vi "Main.vi"() -> ()   [LabVIEW 2015]
doc: "The myRIO Project template acquires acceleration data from the onboard accelerometer and displays the changes of acceleration values in a waveform chart."
uses:
  <vilib>/myRIO/Common/Instrument Driver Framework/myRIO v1.0/Encoder/typedefs/Encoder Signal Mode.ctl
  <vilib>/myRIO/Instrument Drivers/Onboard IO/Encoder/typedefs/Encoder Reference.ctl
  <vilib>/myRIO/Common/Instrument Driver Framework/Utilities/typedefs/myRIO Generic Hardware Reference.ctl
  <vilib>/myRIO/Common/Instrument Driver Framework/Utilities/typedefs/Hardware Version Enum.ctl
  <vilib>/myRIO/Common/Instrument Driver Framework/Utilities/typedefs/myRIO v1.0 Reference.ctl
  <vilib>/myRIO/Common/Instrument Driver Framework/Utilities/typedefs/Generic FPGA Reference.ctl
  <vilib>/myRIO/Common/Instrument Driver Framework/myRIO v1.0/Encoder/typedefs/Encoder Channels Enum.ctl
  <vilib>/myRIO/Common/Instrument Driver Framework/myRIO v1.0/Encoder/typedefs/Encoder Configuration v1.0.ctl
  <vilib>/userdefined/High Color/nirio_resource_hc.ctl
  <vilib>/myRIO/Instrument Drivers/Onboard IO/PWM/typedefs/PWM Reference.ctl
  <vilib>/myRIO/Common/Instrument Driver Framework/myRIO v1.0/PWM/typedefs/PWM Channels Enum.ctl
  <vilib>/myRIO/Instrument Drivers/Onboard IO/PWM/typedefs/PWM Configuration.ctl
  <vilib>/myRIO/Instrument Drivers/Onboard IO/DIO/typedefs/DIO Reference.ctl
  <vilib>/myRIO/Common/Instrument Driver Framework/myRIO v1.0/DIO/typedefs/DIO Channels List.ctl
  <vilib>/myRIO/Common/Instrument Driver Framework/myRIO v1.0/DIO/typedefs/DIO Channels Enum.ctl
  <vilib>/myRIO/Common/Instrument Driver Framework/Utilities/vis/Is FPGA Ref Available.vi
  <vilib>/myRIO/Common/Instrument Driver Framework/myRIO v1.0/Encoder/vis/myRIO v1.1 Open Encoder.vi
  <vilib>/myRIO/Instrument Drivers/Onboard IO/Encoder/vis/Read.vi
  <vilib>/myRIO/Common/Instrument Driver Framework/myRIO v1.0/PWM/vis/myRIO v1.1 Open PWM.vi
  <vilib>/myRIO/Instrument Drivers/Onboard IO/PWM/vis/Set Duty Cycle and Frequency.vi
  <vilib>/myRIO/Common/Instrument Driver Framework/myRIO v1.0/DIO/vis/myRIO v1.1 Open DIO.vi
  <vilib>/myRIO/Instrument Drivers/Onboard IO/DIO/vis/Write.vi
  <vilib>/myRIO/Common/Instrument Driver Framework/Utilities/vis/Validate Channels.vi
  <vilib>/myRIO/Common/Instrument Driver Framework/myRIO v1.0/Encoder/vis/myRIO v1.0 Reserve Encoder.vi
  <vilib>/myRIO/Common/Instrument Driver Framework/myRIO v1.0/PWM/vis/myRIO v1.0 Reserve PWM.vi
  <vilib>/myRIO/Common/Instrument Driver Framework/myRIO v1.0/DIO/vis/myRIO v1.0 Reserve DIO.vi
  <vilib>/myRIO/Common/Instrument Driver Framework/myRIO v1.0/UART/vis/myRIO v1.0 Close UART.vi
  <vilib>/myRIO/Common/Instrument Driver Framework/myRIO v1.0/Encoder/vis/myRIO v1.0 Build MUX Configuration Encoder.vi
  <vilib>/myRIO/Common/Instrument Driver Framework/myRIO v1.0/Resource Manager/vis/myRIO v1.0 Reserve Channel List.vi
  <vilib>/myRIO/Common/Instrument Driver Framework/myRIO v1.0/PWM/vis/myRIO v1.0 Build MUX Configuration PWM.vi
  <vilib>/myRIO/Common/Instrument Driver Framework/myRIO v1.0/DIO/vis/myRIO v1.0 Build MUX Configuration DIO.vi
  <vilib>/myRIO/Common/Instrument Driver Framework/myRIO v1.0/Resource Manager/vis/myRIO v1.0 Create Configuration List.vi
  <vilib>/myRIO/Common/Instrument Driver Framework/myRIO v1.0/Resource Manager/vis/myRIO v1.0 Reserve Channel.vi
  <vilib>/myRIO/Common/Instrument Driver Framework/myRIO v1.0/Resource Manager/vis/myRIO v1.0 Unreserve Channel.vi
  <vilib>/myRIO/Common/Instrument Driver Framework/myRIO v1.0/Resource Manager/vis/myRIO v1.0 Build Mutex Name.vi
  <vilib>/Utility/VariantDataType/GetNumericInfo.vi
  <vilib>/Utility/error.llb/Error Cluster From Error Code.vi
  <vilib>/myRIO/Common/Instrument Driver Framework/myRIO v1.0/myRIO v1.1 Open.vi
  <vilib>/myRIO/Common/Instrument Driver Framework/Utilities/vis/IO Manager.vi
  <vilib>/myRIO/Common/Instrument Driver Framework/Utilities/vis/Configuration Manager.vi
  <vilib>/myRIO/Common/Instrument Driver Framework/myRIO v1.0/Resource Manager/vis/myRIO v1.0 Configure IO.vi
  <vilib>/myRIO/Common/Instrument Driver Framework/myRIO v1.0/myRIO v1.0 Close.vi
  <vilib>/myRIO/Common/Instrument Driver Framework/myRIO v1.0/Encoder/vis/myRIO v1.0 Configure Encoder.vi
  <vilib>/myRIO/Common/Instrument Driver Framework/myRIO v1.0/Encoder/vis/myRIO v1.0 Read Encoder.vi
  <vilib>/myRIO/Common/Instrument Driver Framework/myRIO v1.0/PWM/vis/myRIO v1.0 Write PWM.vi
  <vilib>/myRIO/Common/Instrument Driver Framework/myRIO v1.0/DIO/vis/myRIO v1.0 Write DIO.vi
  <vilib>/myRIO/Common/Instrument Driver Framework/Utilities/vis/FPGA Ref Manager.vi
  <vilib>/myRIO/Common/Instrument Driver Framework/myRIO v1.0/myRIO v1.0 Reset FPGA.vi
  <vilib>/myRIO/Common/Instrument Driver Framework/myRIO v1.0/IRQ/vis/myRIO v1.0 IRQ Info FGV.vi
  <vilib>/myRIO/Common/Instrument Driver Framework/myRIO v1.0/IRQ/vis/myRIO v1.0 Timer IRQ Info FGV.vi
  <vilib>/myRIO/Common/Instrument Driver Framework/myRIO v1.0/IRQ/vis/myRIO v1.0 ISR Agent.vi
  <vilib>/myRIO/Express VI/Onboard IO/Encoder/Encoder Express VI.xnode
  <vilib>/myRIO/Common/Instrument Driver Framework/myRIO v1.0/Encoder/typedefs/Encoder Count Direction Enum.ctl
  <vilib>/myRIO/Instrument Drivers/Onboard IO/Encoder/vis/myRIO Encoder Open.xnode
  <vilib>/myRIO/Express VI/Onboard IO/PWM/PWM Express VI.xnode
  <vilib>/myRIO/Instrument Drivers/Onboard IO/PWM/vis/myRIO PWM Open.xnode
  <vilib>/myRIO/Express VI/Onboard IO/DO/DO Express VI.xnode
  <vilib>/myRIO/Instrument Drivers/Onboard IO/DIO/vis/myRIO DIO Open.xnode
  <vilib>/myRIO/Instrument Drivers/Utilities/Utilities.lvlib
  <vilib>/myRIO/Instrument Drivers/Onboard IO/Encoder/Encoder.lvlib
  <vilib>/myRIO/Instrument Drivers/Onboard IO/DIO/DIO.lvlib
  <vilib>/myRIO/Instrument Drivers/Onboard IO/PWM/PWM.lvlib
panel:
  in  "Up/Down control":bool
  out "PWM":dbl(graph)
  in  "K4":dbl
  in  "K3":dbl
  in  "K2":dbl
  in  "K1":dbl
  in  "Stop Button":bool
  out "Gauge":dbl(knob) scale=0.0..360.0
  in  "ON OFF":bool
  out "x >= 0?":bool
  out ".not. x?":bool
  out "abs(x)":dbl
  out "filtTheta":dbl
  out "Theta control 2":dbl
  out "Theta control":dbl
  out "Control":bool
  out "dPhi":dbl(graph)
  out "dTheta":dbl(graph)
  in  "Swing up gain":dbl
  out "Rad dPhi":dbl
  out "Rad Theta":dbl
  out "Rad Phi":dbl
  out "Direction Motor":dbl
  out "Counter Motor":dbl
  out "error out":errorcluster
  # "Overview: The myRIO Project template acquires acceleration data from the onboard accelerometer and displays the changes of acceleration values in a waveform chart.\nInstructions:\n1. Check the myRIO target IP address in the project and make sure the target IP address is correct. \n2. Run this VI."
types:
  T1 = typedef "Encoder.lvlib/Encoder Reference.ctl" = cluster{"myRIO Reference":T2, "Encoder Channels Enum":T6}
  T2 = typedef "myRIO Generic Hardware Reference.ctl" = cluster{"myRIO Model":T3, "myRIO Hardware Reference":T4}
  T3 = typedef "Hardware Version Enum.ctl" = enum16{"Unknown", "myRIO-1900", "myRIO-1950", "roboRIO"}
  T4 = typedef "myRIO v1.0 Reference.ctl" = cluster{"Generic FPGA Reference":T5, "Allow multiple opens":bool}
  T5 = typedef "Generic FPGA Reference.ctl" = refnum<k20>
  T6 = typedef "Encoder Channels Enum.ctl" = enum16{"Not Connected", "C/ENC0", "C/ENC1", "A/ENC", "B/ENC", "DIO/ENC0", "DIO/ENC1", "DIO/ENC2", "DIO/ENC3", "DIO/ENC4"}
  T7 = typedef "Encoder Signal Mode.ctl" = enum16{"Quadrature phase signal", "Step and direction signal"}
  T8 = typedef "nirio_resource_hc.ctl" = tag
  T9 = typedef "DIO.lvlib/DIO Reference.ctl" = cluster{"myRIO Reference":T2, "DIO Channels List":T10}
  T10 = typedef "DIO Channels List.ctl" = T11[]
  T11 = typedef "DIO Channels Enum.ctl" = enum16{"Not Connected", "C/DIO0", "C/DIO1", "C/DIO2", "C/DIO3", "C/DIO4", "C/DIO5", "C/DIO6", "C/DIO7", "A/DIO0", "A/DIO1", "A/DIO2", "A/DIO3", "A/DIO4", "A/DIO5", "A/DIO6", "A/DIO7", "A/DIO8", "A/DIO9", "A/DIO10", "A/DIO11", "A/DIO12", "A/DIO13", "A/DIO14", "A/DIO15", "B/DIO0", "B/DIO1", "B/DIO2", "B/DIO3", "B/DIO4", "B/DIO5", "B/DIO6", "B/DIO7", "B/DIO8", "B/DIO9", "B/DIO10", "B/DIO11", "B/DIO12", "B/DIO13", "B/DIO14", "B/DIO15", "LED0", "LED1", "LED2", "LED3", "Button0", "DIO/DIO0", "DIO/DIO1", "DIO/DIO2", "DIO/DIO3", "DIO/DIO4", "DIO/DIO5", "DIO/DIO6", "DIO/DIO7", "DIO/DIO8", "DIO/DIO9", "SPI/CS0", "SPI/CS1", "SPI/CS2", "SPI/CS3", "LED RADIO (Green)", "LED RADIO (Red)", "LED COMM (Green)", "LED COMM (Red)", "LED MODE (Green)", "LED MODE (Red)"}
  T12 = typedef "PWM.lvlib/PWM Reference.ctl" = cluster{"myRIO Reference":T2, "PWM Channels Enum":T13, "PWM Configuration":T14}
  T13 = typedef "PWM Channels Enum.ctl" = enum16{"Not Connected", "C/PWM0", "C/PWM1", "A/PWM0", "A/PWM1", "A/PWM2", "B/PWM0", "B/PWM1", "B/PWM2", "PWM/PWM0", "PWM/PWM1", "PWM/PWM2", "PWM/PWM3", "PWM/PWM4", "PWM/PWM5", "PWM/PWM6", "PWM/PWM7", "PWM/PWM8", "PWM/PWM9"}
  T14 = typedef "PWM.lvlib/PWM Configuration.ctl" = cluster{"Frequency":dbl, "Duty Cycle":dbl}
  T15 = typedef "Encoder Count Direction Enum.ctl" = enum16{"Counting Up", "Counting Down"}
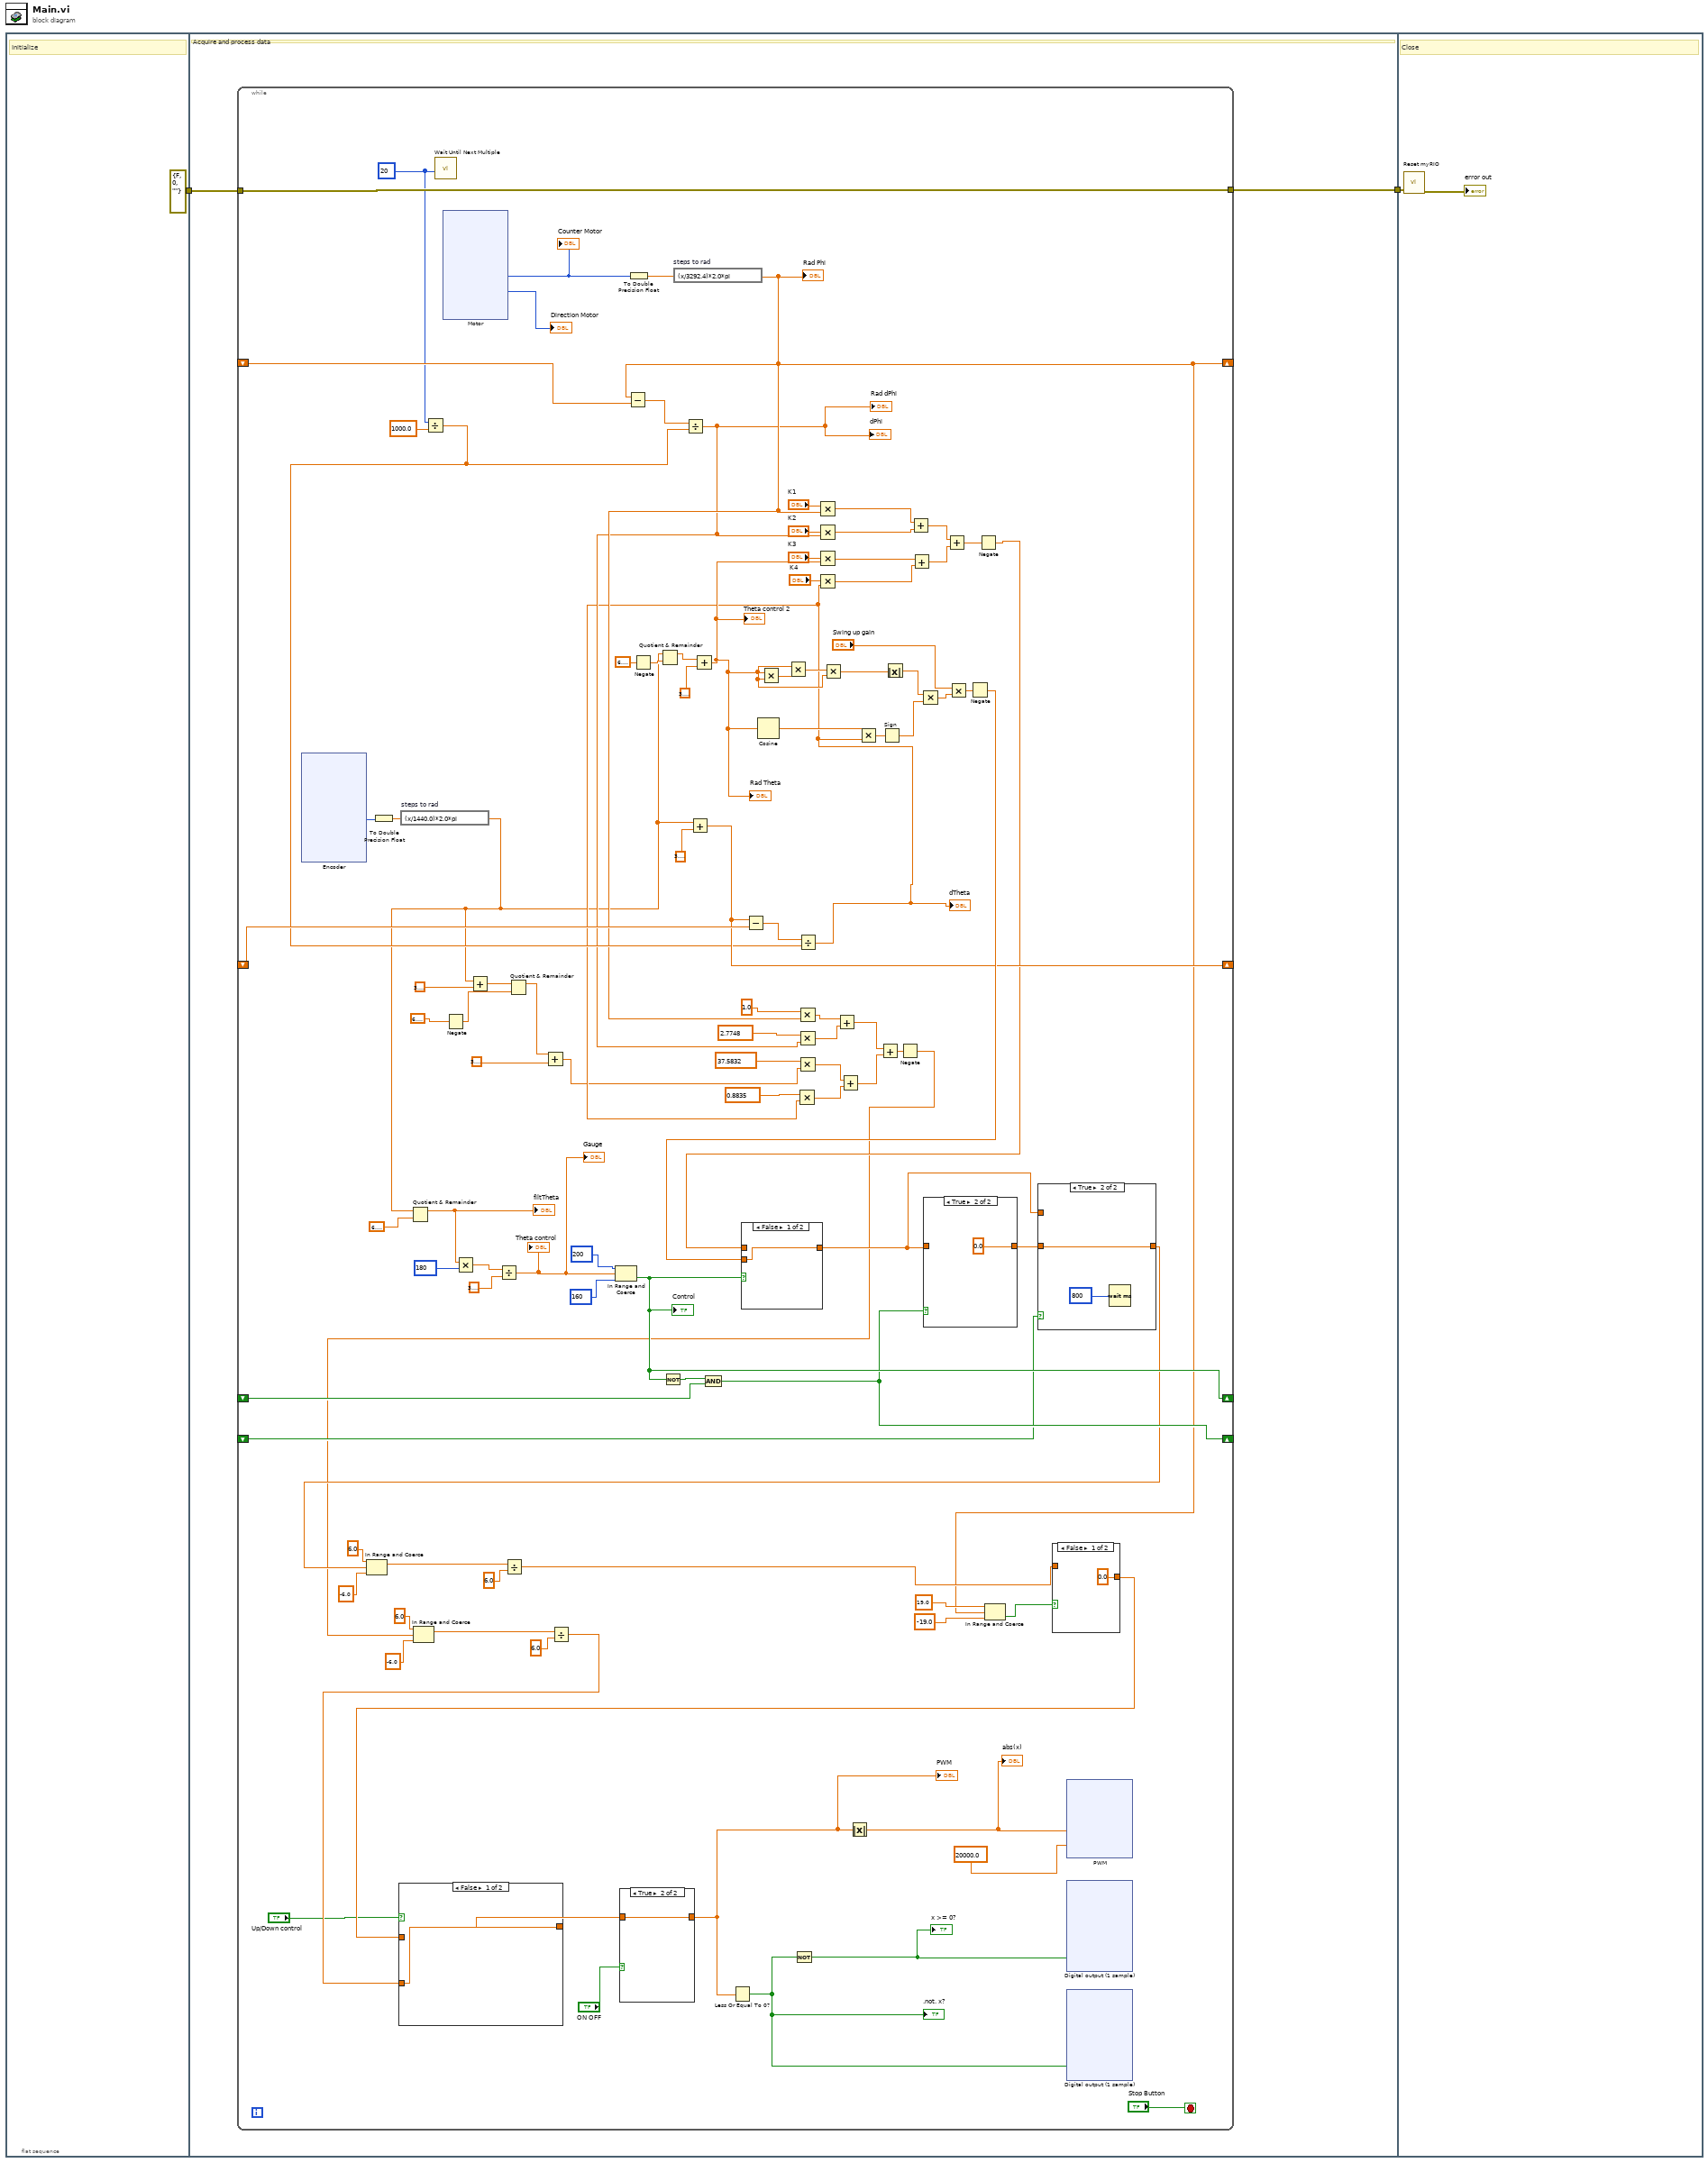
[diagram p0: block diagram]
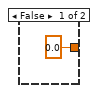
[diagram p3: hidden frame]
diagram:
  n1 = flat-sequence {
    tunnel: [errorcluster {"status"=FALSE, "code"=0, "source"=""} ("error in (no error)")] -> w2
    tunnel: w2 -> [w4]
    tunnel: [w5] -> w1
    tunnel: w1 -> [w322]
    frame #0 {
      # "Initialize"
    }
    frame #1 {
      # "Acquire and process data"
      n2 = while {
        tunnel: w4 -> [w105]
        tunnel: [w105] -> w5
        shift-right: [w38] -> _
        shift-left: _ -> [w104]
        shift-right: [w52] -> _
        shift-left: _ -> [w53]
        shift-right: [w64] -> _
        shift-left: _ -> [w63]
        shift-right: [w62] -> _
        shift-left: _ -> [w61]
        stop <- "Stop Button" stop-if-true
        w66 = u32 20 ("Count(mSec)")
        n3 = xnode "Encoder"() -> ("Counter Value"=w50:i32)  [unwired: 2 in, 3 out]
        n4 = To Double Precision Float(number=w50) -> (double precision float=w108:dbl)
        n5 = expression code="(x/1440.0)*2.0*pi" "steps to rad"(w108) -> (w23:dbl)
        n6 = Quotient & Remainder(x=w23, y=6.283185307179586) -> (x-y*floor(x/y)=w82:dbl)  [unwired: 1 out]
        "filtTheta" <- w82
        n7 = Divide(x=w66, y=1000.0) -> (x/y=w51:dbl)
        n8 = call "Wait Until Next Multiple"("Count(mSec)"=w66) -> ()  [unwired: 1 out]
        n9 = xnode "Motor"() -> ("Counter Value"=w109:i32, "Counter Direction"=→"Direction Motor":T15)  [unwired: 2 in, 2 out]
        "Counter Motor" <- w109
        n10 = Negate(x=6.283185307179586) -> (-x=w20:dbl)
        n11 = Multiply(x=w82, y=180) -> (x*y=w80:dbl)
        n12 = Add(x=w23, y=3.141592653589793) -> (x+y=w19:dbl)
        n13 = Divide(x=w80, y=3.141592653589793) -> (x/y=w55:dbl)
        "Theta control" <- w55
        "Gauge" <- w55
        n14 = Quotient & Remainder(x=w19, y=w20) -> (x-y*floor(x/y)=w17:dbl)  [unwired: 1 out]
        n15 = Add(x=w17, y=3.141592653589793) -> (x+y=w16:dbl)
        n16 = In Range and Coerce(upper limit=200, x=w55, lower limit=160) -> (In Range?=w64:bool)  [unwired: 1 out]
        "Control" <- w64
        n17 = To Double Precision Float(number=w109) -> (double precision float=w107:dbl)
        n18 = Negate(x=6.283185307179586) -> (-x=w71:dbl)
        n19 = Quotient & Remainder(x=w23, y=w71) -> (x-y*floor(x/y)=w72:dbl)  [unwired: 1 out]
        n20 = Not(x=w64) -> (.not. x?=w65:bool)
        n21 = expression code="(x/3292.4)*2.0*pi" "steps to rad"(w107) -> (w38:dbl)
        "Rad Phi" <- w38
        n22 = Subtract(x=w38, y=w104) -> (x-y=w103:dbl)
        n23 = Divide(x=w103, y=w51) -> (x/y=w37:dbl)
        "Rad dPhi" <- w37
        "dPhi" <- w37
        n24 = Add(x=w23, y=3.141592653589793) -> (x+y=w52:dbl)
        n25 = Add(x=w72, y=3.141592653589793) -> (x+y=w69:dbl)
        "Rad Theta" <- w69
        "Theta control 2" <- w69
        n26 = And(x=w65, y=w63) -> (x .and. y?=w62:bool)
        n27 = Subtract(x=w52, y=w53) -> (x-y=w102:dbl)
        n28 = Cosine(x=w69) -> (cos(x)=w100:dbl)
        n29 = Multiply(x=w69, y=w69) -> (x*y=w93:dbl)
        n30 = Multiply(x=w69, y=w93) -> (x*y=w70:dbl)
        n31 = Multiply(x=1.0, y=w38) -> (x*y=w35:dbl)
        n32 = Multiply(x=2.7748, y=w37) -> (x*y=w34:dbl)
        n33 = Multiply(x=37.5832, y=w16) -> (x*y=w33:dbl)
        n34 = Divide(x=w102, y=w51) -> (x/y=w36:dbl)
        "dTheta" <- w36
        n35 = Multiply(x=0.8835, y=w36) -> (x*y=w32:dbl)
        n36 = Multiply(x="K1", y=w38) -> (x*y=w84:dbl)
        n37 = Multiply(x="K2", y=w37) -> (x*y=w85:dbl)
        n38 = Multiply(x="K3", y=w69) -> (x*y=w86:dbl)
        n39 = Multiply(x="K4", y=w36) -> (x*y=w87:dbl)
        n40 = Multiply(x=w70, y=w69) -> (x*y=w68:dbl)
        n41 = Add(x=w35, y=w34) -> (x+y=w31:dbl)
        n42 = Add(x=w33, y=w32) -> (x+y=w30:dbl)
        n43 = Multiply(x=w100, y=w36) -> (x*y=w99:dbl)
        n44 = Add(x=w31, y=w30) -> (x+y=w15:dbl)
        n45 = Sign(1:w99) -> (0:w101:dbl)
        n46 = Absolute Value(x=w68) -> (abs(x)=w94:dbl)
        n47 = Negate(x=w15) -> (-x=w10:dbl)
        n48 = In Range and Coerce(upper limit=6.0, x=w10, lower limit=-6.0) -> (coerced(x)=w12:dbl)  [unwired: 1 out]
        n49 = Divide(x=w12, y=6.0) -> (x/y=w9:dbl)
        n50 = Add(x=w84, y=w85) -> (x+y=w89:dbl)
        n51 = Add(x=w86, y=w87) -> (x+y=w88:dbl)
        n52 = Multiply(x=w94, y=w101) -> (x*y=w92:dbl)
        n53 = Add(x=w89, y=w88) -> (x+y=w45:dbl)
        n54 = Multiply(x="Swing up gain", y=w92) -> (x*y=w83:dbl)
        n55 = Negate(x=w83) -> (-x=w58:dbl)
        n56 = Negate(x=w45) -> (-x=w44:dbl)
        n57 = case shown="False" w64 {
          tunnel: w44 -> [_ w237]
          tunnel: w58 -> [w236 _]
          tunnel: [w236 w237] -> w59
          frame False {
          }
          frame True {
          }
        }
        n58 = case shown="True" w62 {
          tunnel: w59 -> [w234 _]
          tunnel: [w234 0.0] -> w60
          frame False {
          }
          frame True {
          }
        }
        n59 = In Range and Coerce(upper limit=19.0, x=w38, lower limit=-19.0 ("upper limit")) -> (In Range?=w95:bool)  [unwired: 1 out]
        n60 = case shown="True" w61 {
          tunnel: w60 -> [_ w232]
          tunnel: [w231 w232] -> w43
          tunnel: w59 -> [w231 _]
          frame False {
          }
          frame True {
            n61 = Wait (ms)(milliseconds to wait=u32 800) -> ()  [unwired: 1 out]
          }
        }
        n62 = In Range and Coerce(upper limit=6.0, x=w43, lower limit=-6.0) -> (coerced(x)=w42:dbl)  [unwired: 1 out]
        n63 = Divide(x=w42, y=6.0) -> (x/y=w40:dbl)
        n64 = case shown="False" w95 {
          tunnel: [0.0 ("upper limit") w239] -> w29
          tunnel: w40 -> [_ w239]
          frame False {
          }
          frame True {
          }
        }
        n65 = case shown="False" "Up/Down control" {
          tunnel: w29 -> [_ w112]
          tunnel: [w111 w112] -> w28
          tunnel: w9 -> [w111 _]
          frame False {
          }
          frame True {
          }
        }
        n66 = case shown="True" "ON OFF" {
          tunnel: [0.0 w160] -> w7
          tunnel: w28 -> [_ w160]
          frame False {
          }
          frame True {
          }
        }
        "PWM" <- w7
        n67 = Less Or Equal To 0?(x=w7) -> (x <= 0?=w39:bool)
        ".not. x?" <- w39
        n68 = Not(x=w39) -> (.not. x?=w57:bool)
        "x >= 0?" <- w57
        n69 = Absolute Value(x=w7) -> (abs(x)=w8:dbl)
        "abs(x)" <- w8
        n70 = xnode "PWM"("Duty Cycle"=w8, "Frequency [Hz]"=20000.0) -> ()  [unwired: 1 in, 1 out]
        n71 = xnode "Digital output (1 sample)"("A/DIO8 (Pin 27)"=w57) -> ()  [unwired: 1 in, 1 out]
        n72 = xnode "Digital output (1 sample)"("A/DIO9 (Pin 29)"=w39) -> ()  [unwired: 1 in, 1 out]
      }
    }
    frame #2 {
      # "Close"
      n73 = call <vilib>:"Reset myRIO.vi"("error in (no error)"=w322) -> ("error out"=→"error out":errorcluster)  [unwired: 10 in]
    }
  }
